vi "ReleaseStringQueue.vi"(8 "error in":errorcluster, 11 "QueueIn":variant) -> (0 "错误输出":errorcluster caption="error out")   [LabVIEW 2013]
panel:
  in  "queue out":refnum<queue>
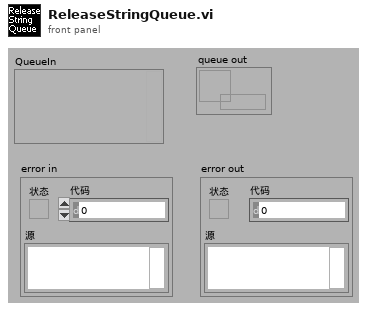
[diagram p1: front panel]
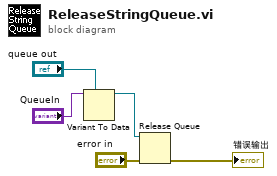
[diagram p0: block diagram]
diagram:
  n1 = Variant To Data(type="queue out", Variant="QueueIn") -> (data=w2:refnum<queue>)  [unwired: 1 in, 1 out]
  n2 = Release Queue(queue=w2, error in (no error)="error in") -> (error out=→"错误输出":errorcluster)  [unwired: 3 out]
